vi "Write Last BG Loop.vi"(8 "error in (no error)":errorcluster, 10 "Last BG Loop":i32, 11 "Worker Actor in":refnum<class "Worker Actor.lvclass">) -> (0 "error out":errorcluster, 3 "Worker Actor out":refnum<class "Worker Actor.lvclass">)   [LabVIEW 2021, in "Worker Actor.lvclass"]
uses:
  Worker Actor.lvclass
  Worker Actor.lvclass/Worker Actor.ctl
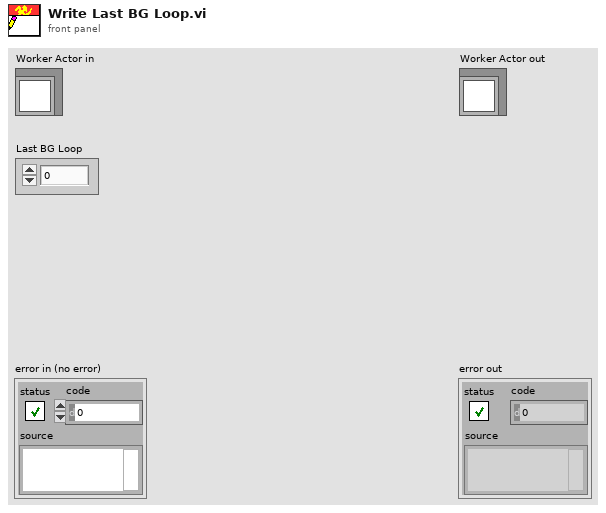
[diagram p1: front panel]
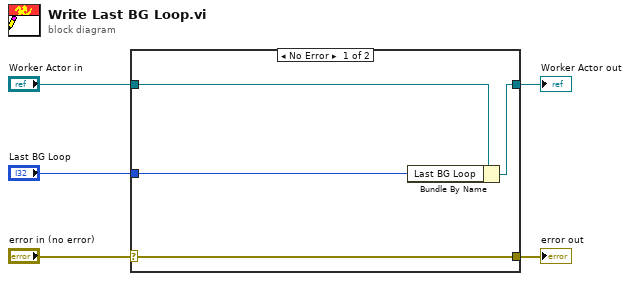
[diagram p0: block diagram]
diagram:
  n1 = case shown="No Error" "error in (no error)" {
    selector: "error in (no error)" -> [w9 w10]
    tunnel: [w9 w10] -> w4
    tunnel: [w7 w11] -> w2
    tunnel: "Worker Actor in" -> [w8 w11]
    tunnel: "Last BG Loop" -> [w6 _]
    frame No Error {
      n2 = Bundle By Name(cluster=w8, "Last BG Loop"=w6) -> (w7:refnum<class "Worker Actor.lvclass">)
    }
    frame Error {
    }
  }
  "error out" <- w4
  "Worker Actor out" <- w2
